vi "OutBitsPrepareForScan.vi"() -> (2 "listeningWorks":bool)   [LabVIEW 2014]
uses:
  OutbitsStateControl.ctl
  <vilib>/rvi/Emulation/niFpgaGetClockAttributes.vi
  <vilib>/rvi/Emulation/niFpgaSctlEmulationGetInTimedLoop.vi
  <vilib>/rvi/Emulation/niFpgaEmulationReportErrorSimple.vi
  OutbitsGlobalVars.vi
  Sequencer/sequencerGlobVars.vi
  <vilib>/rvi/Emulation/niFpgaCriticalErrorInLSC.vi
panel:
  # "prepare the outbits module for a scan by\n setting the stoplistening flag to false and\n setting the cmd to loading"
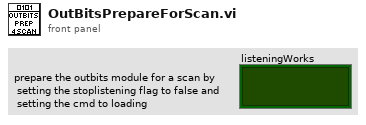
[diagram p1: front panel]
types:
  T1 = typedef "OutbitsStateControl.ctl" = enum16{"Init", "Idle", "loading", "listening", "clearing", "error"}
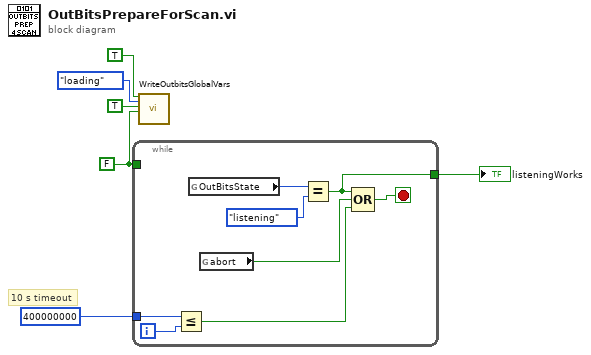
[diagram p0: block diagram]
diagram:
  w5 = FALSE ("OutBitStopListening")
  # "10 s timeout"
  n1 = while {
    tunnel: w5 -> [_]
    tunnel: [w10] -> w2
    tunnel: 400000000 ("x") -> [w8]
    i -> [w9]
    stop <- w12 stop-if-true
    n2 = Less Or Equal?(x=w8, y=w9) -> (x <= y?=w7:bool)
    n3 = global read "OutbitsGlobalVars.vi" "OutBitsState"() -> (w14:T1)
    n4 = global read "sequencerGlobVars.vi" "abort"() -> (w11:bool)
    n5 = Equal?(x=w14, y=OutbitsStateControl."listening" ("OutBitsState")) -> (x = y?=w10:bool)
    n6 = Compound Arithmetic op=OR(w10, w11, w7) -> (w12:bool)
  }
  "listeningWorks" <- w2
  n7 = call "WriteOutbitsGlobalVars.vi"("writeState"=TRUE, "OutBitsState"=OutbitsStateControl."loading", "write_OutBitStopListening"=TRUE, "OutBitStopListening"=w5) -> ()  [unwired: 15 in, 1 out]
